vi "VolumeDataExtract.vi"(8 "error in (no error)":errorcluster, 11 "VolumeRawData":dbl[][](array[numeric])) -> (0 "error out":errorcluster)   [LabVIEW 2017]
panel:
  out "VolumePlanesData":dbl[][][][](array[numeric])
  in  "number of pixels in a miniscan":i32
  in  "number of miniscans in a Plane":i32
  in  "number of planes":i32
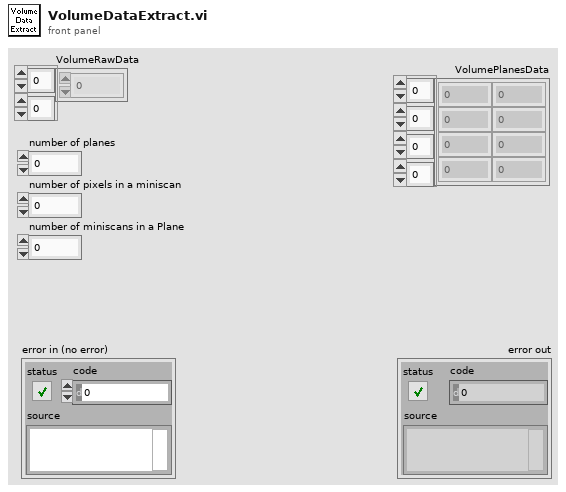
[diagram p1: front panel]
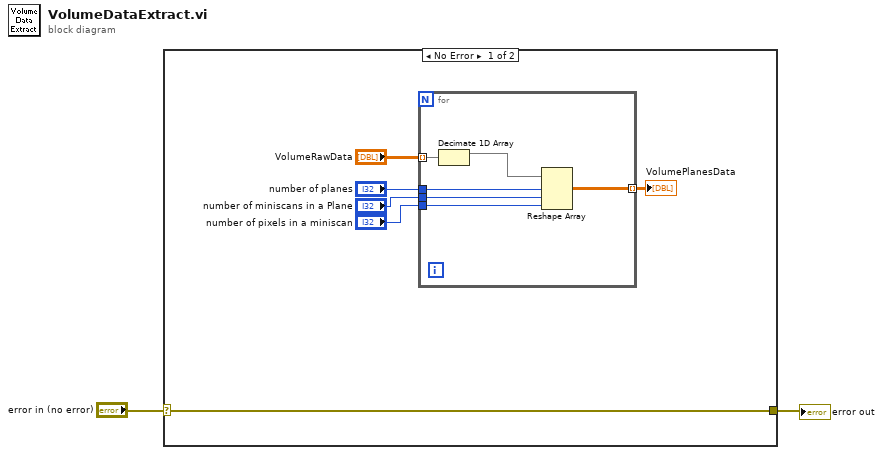
[diagram p0: block diagram]
diagram:
  n1 = case shown="No Error" "error in (no error)" {
    selector: "error in (no error)" -> [w4 w15]
    tunnel: [w4 w15] -> w1
    frame No Error {
      n2 = for {
        tunnel: "VolumeRawData" -> [w14] mode=indexing
        tunnel: "number of pixels in a miniscan" -> [w13]
        tunnel: "number of miniscans in a Plane" -> [w12]
        tunnel: "number of planes" -> [w11]
        tunnel: [w9] -> w3 mode=indexing
        n3 = Decimate 1D Array(w14) -> (w10:dbl[])  [unwired: 1 out]
        n4 = Reshape Array(w10, w11, w12, w13) -> (w9:dbl[][][])
      }
      "VolumePlanesData" <- w3
    }
    frame Error {
    }
  }
  "error out" <- w1
